vi "IndexCluster (VData_Index_Name).vi"(11 "variant (destination)":variant) -> (0 "index Array":i32[][](array[numeric]), 1 "Array of VData":variant[](array[variant]), 2 "Names (Array)":string[](array[string]), 3 "variant (destination)out":variant)   [LabVIEW 2011]
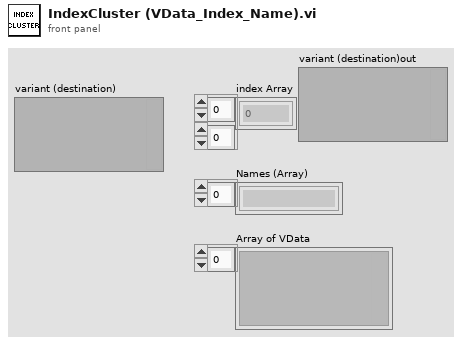
[diagram p1: front panel]
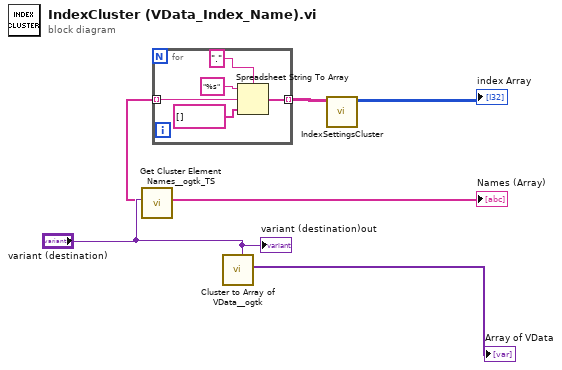
[diagram p0: block diagram]
diagram:
  n1 = call "Get Cluster Element Names__ogtk_TS.vi"("Variant"="variant (destination)") -> ("Names (Array)"=w2:string[])  [unwired: 9 in, 1 out]
  "Names (Array)" <- w2
  n2 = for {
    tunnel: w2 -> [w7] mode=indexing
    tunnel: [w6] -> w1 mode=indexing
    n3 = Spreadsheet String To Array(delimiter (Tab)=".", format string="%s", spreadsheet string=w7, array type (2D Dbl)=string[] []) -> (array=w6:string[])
  }
  n4 = call "Cluster to Array of VData__ogtk.vi"("Cluster"="variant (destination)") -> ("Array of VData"=→"Array of VData":variant[])  [unwired: 9 in, 1 out]
  n5 = call "IndexSettingsCluster.vi"("Names Array"=w1) -> ("index Array"=→"index Array":i32[][])  [unwired: 10 in]
  "variant (destination)out" <- "variant (destination)"
